vi "Configure Voltage Limits.vi"(6 "Low Voltage Limit (-5 V)":dbl=-5.0, 7 "High Voltage Limit (5 V)":dbl=5.0, 8 "error in (no error)":errorcluster, 9 "Enable Voltage Limit (T: Enable)":bool=TRUE, 10 "Channel (1: 1)":i32(ring)=1 items=["1"=1, "2"=2], 11 "VISA resource name":refnum<visa-resource-name>) -> (0 "error out":errorcluster, 3 "VISA resource name out":refnum<visa-resource-name>)   [LabVIEW 2013, in "Agilent 3352X Series.lvlib"]
doc: "Enables and sets the high and low limit voltages for the voltage level settings of the specified channel.\n\n<b>Note</b>:\n(1) Use this VI only with other VIs. The high-level VIs automatically incorporate this functionality. \n(2) This VI does not check the instrument status. If you want to check the instrument status, call the Error Query VI at the conclusion of your output configuration."
uses:
  Agilent 3352X Series.lvlib
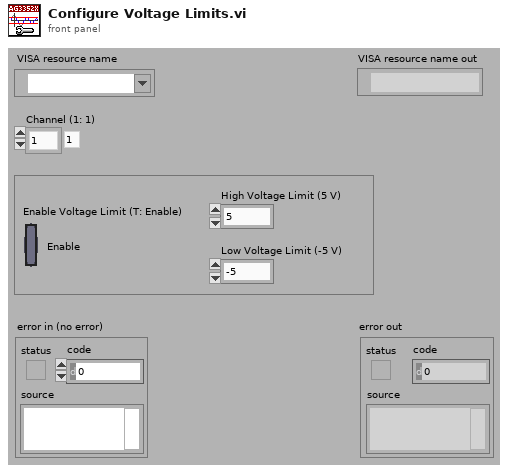
[diagram p1: front panel]
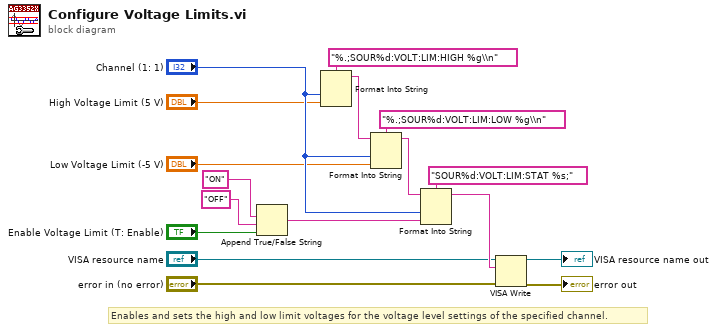
[diagram p0: block diagram]
diagram:
  # "Enables and sets the high and low limit voltages for the voltage level settings of the specified channel."
  n1 = Append True/False String(1:"Enable Voltage Limit (T: Enable)", 2:"OFF", 3:"ON") -> (0:w6:string)  [unwired: 1 out]
  n2 = Format Into String(format string="%.;SOUR%d:VOLT:LIM:HIGH %g\\n", "Channel (1: 1)", "High Voltage Limit (5 V)") -> (resulting string=w14:string)  [unwired: 2 in, 1 out]
  n3 = Format Into String(format string="%.;SOUR%d:VOLT:LIM:LOW %g\\n", initial string=w14, "Channel (1: 1)", "Low Voltage Limit (-5 V)") -> (resulting string=w8:string)  [unwired: 1 in, 1 out]
  n4 = Format Into String(format string="SOUR%d:VOLT:LIM:STAT %s;", initial string=w8, "Channel (1: 1)", w6) -> (resulting string=w5:string)  [unwired: 1 in, 1 out]
  n5 = VISA Write(VISA resource name="VISA resource name", write buffer=w5, error in (no error)="error in (no error)") -> (VISA resource name out=→"VISA resource name out":refnum<visa-resource-name>, error out=→"error out":errorcluster)  [unwired: 1 out]
